vi "Serialize.vi"(8 "error in (no error)":errorcluster, 10 "CI Serializer in":refnum<class "CI Serializer.lvclass">, 11 "Root Node":T1) -> (0 "error out":errorcluster, 2 "CI Serializer out":refnum<class "CI Serializer.lvclass">)   [LabVIEW 2014, in "CI Serializer.lvclass"]
uses:
  CI Serializer.lvclass
  <vilib>/ni/Configuration Framework/Node/NodeRef.ctl
  <vilib>/ni/Configuration Framework/Node/NISE_CEF_Node.lvclass
  Serializable Node/Serializable Node.lvclass
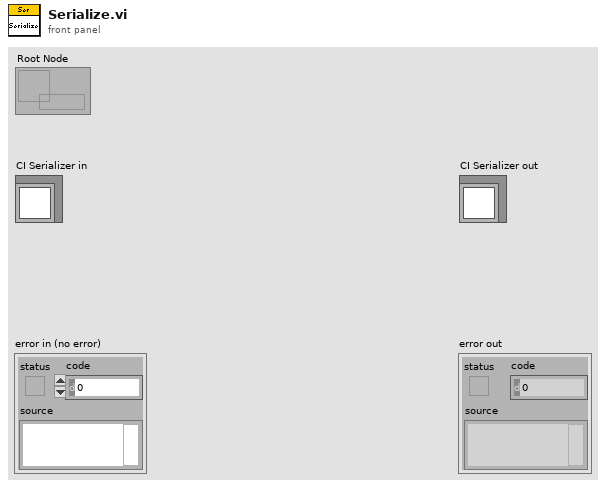
[diagram p1: front panel]
types:
  T1 = typedef "NISE_CEF_Node.lvclass/NodeRef.ctl" = refnum<data-value>
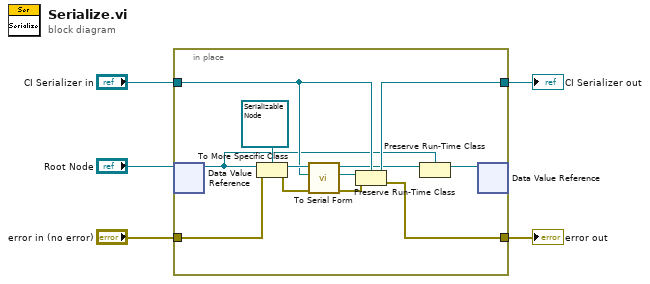
[diagram p0: block diagram]
diagram:
  n1 = in-place {
    in-place-border: "CI Serializer in" -> [w12]
    in-place-border: [w11] -> w3
    in-place-border: "error in (no error)" -> [w10]
    in-place-border: [w6] -> w1
    n2 = in-place-dvr #1("Root Node") -> (w7:refnum<class "NISE_CEF_Node.lvclass">)  [unwired: 1 out]
    n3 = To More Specific Class(target class=refnum<class "Serializable Node.lvclass"> refnum ("Serializable Node in"), reference=w7, error in=w10) -> (specific class reference=w13:refnum<class "Serializable Node.lvclass">, error out=w15:errorcluster)
    n4 = call-dynamic "To Serial Form.vi"("error in (no error)"=w15, "CI Serializer in"=w12, "Serializable Node in"=w13) -> ("error out"=w17:errorcluster, "CI Serializer out"=w16:refnum<class "CI Serializer.lvclass">, "Serializable Node out"=w9:refnum<class "Serializable Node.lvclass">)  [unwired: 5 in, 1 out]
    n5 = Preserve Run-Time Class(object in=w16, error in=w17, 2:w12) -> (object out=w11:refnum<class "CI Serializer.lvclass">, error out=w6:errorcluster)
    n6 = Preserve Run-Time Class(object in=w9, 2:w7) -> (object out=w8:refnum<class "NISE_CEF_Node.lvclass">)  [unwired: 1 in, 1 out]
    n7 = in-place-dvr #1(w8) -> ()  [unwired: 2 out]
  }
  "error out" <- w1
  "CI Serializer out" <- w3
